vi "publish -- get frequency and voltage.vi"(7 "publisher action":T1, 8 "gamma IN (Hz)":dbl=1000.0, 9 "Voltage IN (V)":cdb=1.133070214302279+0.0i, 10 "freq IN (Hz)":dbl=1000.0 format="%#_10f") -> (0 "gamma OUT (Hz)":dbl=1000.0, 1 "Voltage out (V)":cdb=1.133070214302279+0.0i, 2 "freq out (Hz)":dbl=1000.0 format="%#_10f")   [LabVIEW 2018]
uses:
  publisher action.ctl
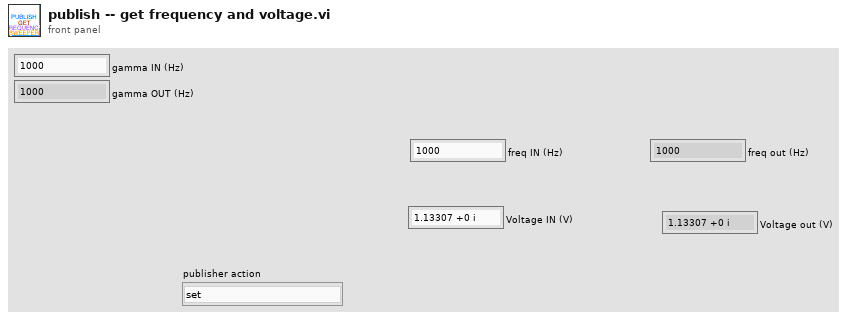
[diagram p1: front panel]
types:
  T1 = typedef "publisher action.ctl" = enum16{"set", "get", "init", "check"}
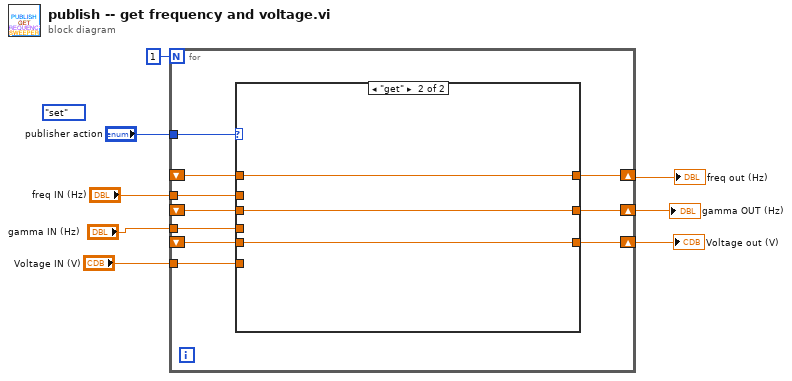
[diagram p0: block diagram]
diagram:
  (unwired) publisher_action."set" ("publisher action")
  n1 = for {
    N: 1 -> [_]
    tunnel: "publisher action" -> [w18]
    tunnel: "freq IN (Hz)" -> [w16]
    shift-right: [w17] -> w4
    shift-left: _ -> [w15]
    shift-right: [w14] -> w3
    shift-left: _ -> [w12]
    tunnel: "Voltage IN (V)" -> [w13]
    tunnel: "gamma IN (Hz)" -> [w11]
    shift-right: [w10] -> w1
    shift-left: _ -> [w9]
    n2 = case shown="\"get\"" w18 {
      tunnel: [w21 w24] -> w17
      tunnel: w16 -> [w21 _]
      tunnel: w15 -> [_ w24]
      tunnel: [w20 w23] -> w14
      tunnel: w13 -> [w20 _]
      tunnel: w12 -> [_ w23]
      tunnel: w11 -> [w19 _]
      tunnel: [w19 w22] -> w10
      tunnel: w9 -> [_ w22]
      frame "set", Default {
      }
      frame "get" {
      }
    }
  }
  "Voltage out (V)" <- w3
  "freq out (Hz)" <- w4
  "gamma OUT (Hz)" <- w1
